vi "iPSset.vi"(7 "Field Rate, T/min":dbl, 8 "error in (no error)":errorcluster, 9 "Target Field, T":dbl, 10 "iPSSetCtrl":T1, 11 "VISA resource name":refnum<visa-resource-name>) -> (0 "error out":errorcluster, 1 "read buffer":string, 2 "number":dbl, 3 "VISA resource name out":refnum<visa-resource-name>)   [LabVIEW 2017]
uses:
  controls/iPSsetCtrl.ctl
  <vilib>/regexp/Match Regular Expression.xnode
panel:
  out "call chain":string[](array[string])
  out "concatenated string 2":string
  out "concatenated string":string
  out "after match":string
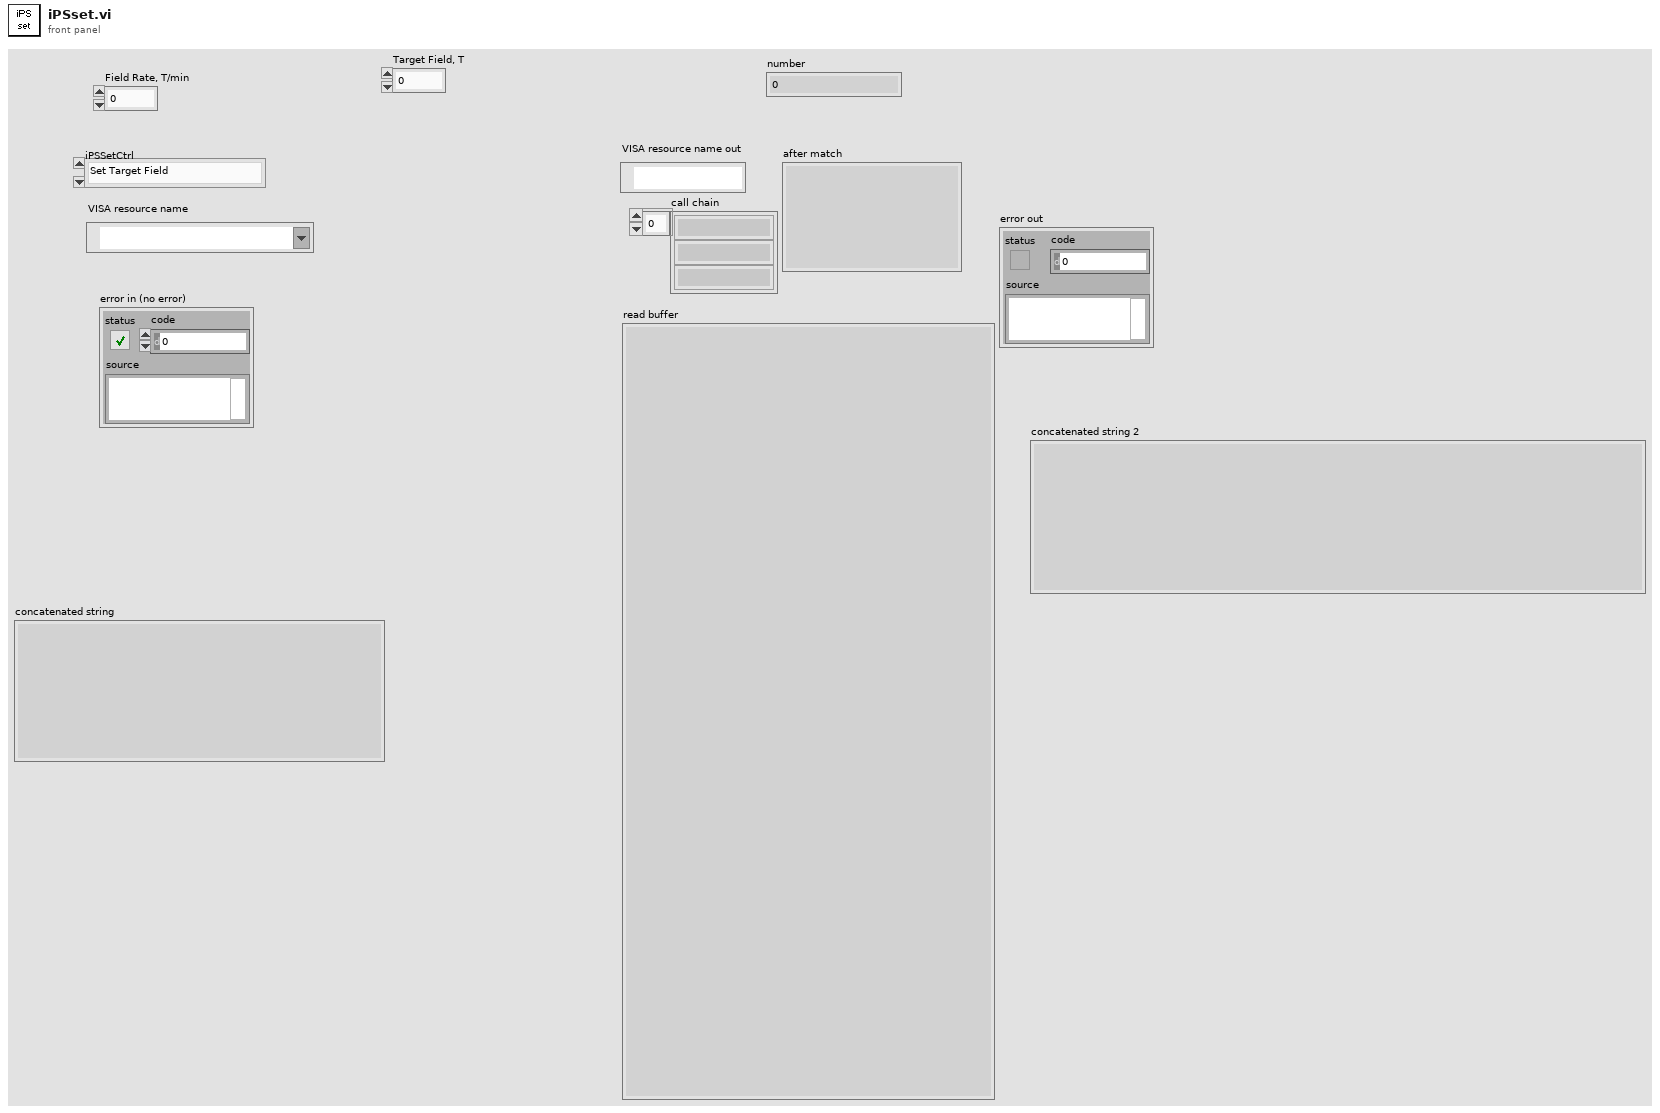
[diagram p1: front panel]
types:
  T1 = typedef "iPSsetCtrl.ctl" = enum16{"Set Target Field", "Set Target Field Rate", "Switch Heater ON", "Switch Heater OFF", "Go to Field", "Go to Zero", "Hold"}
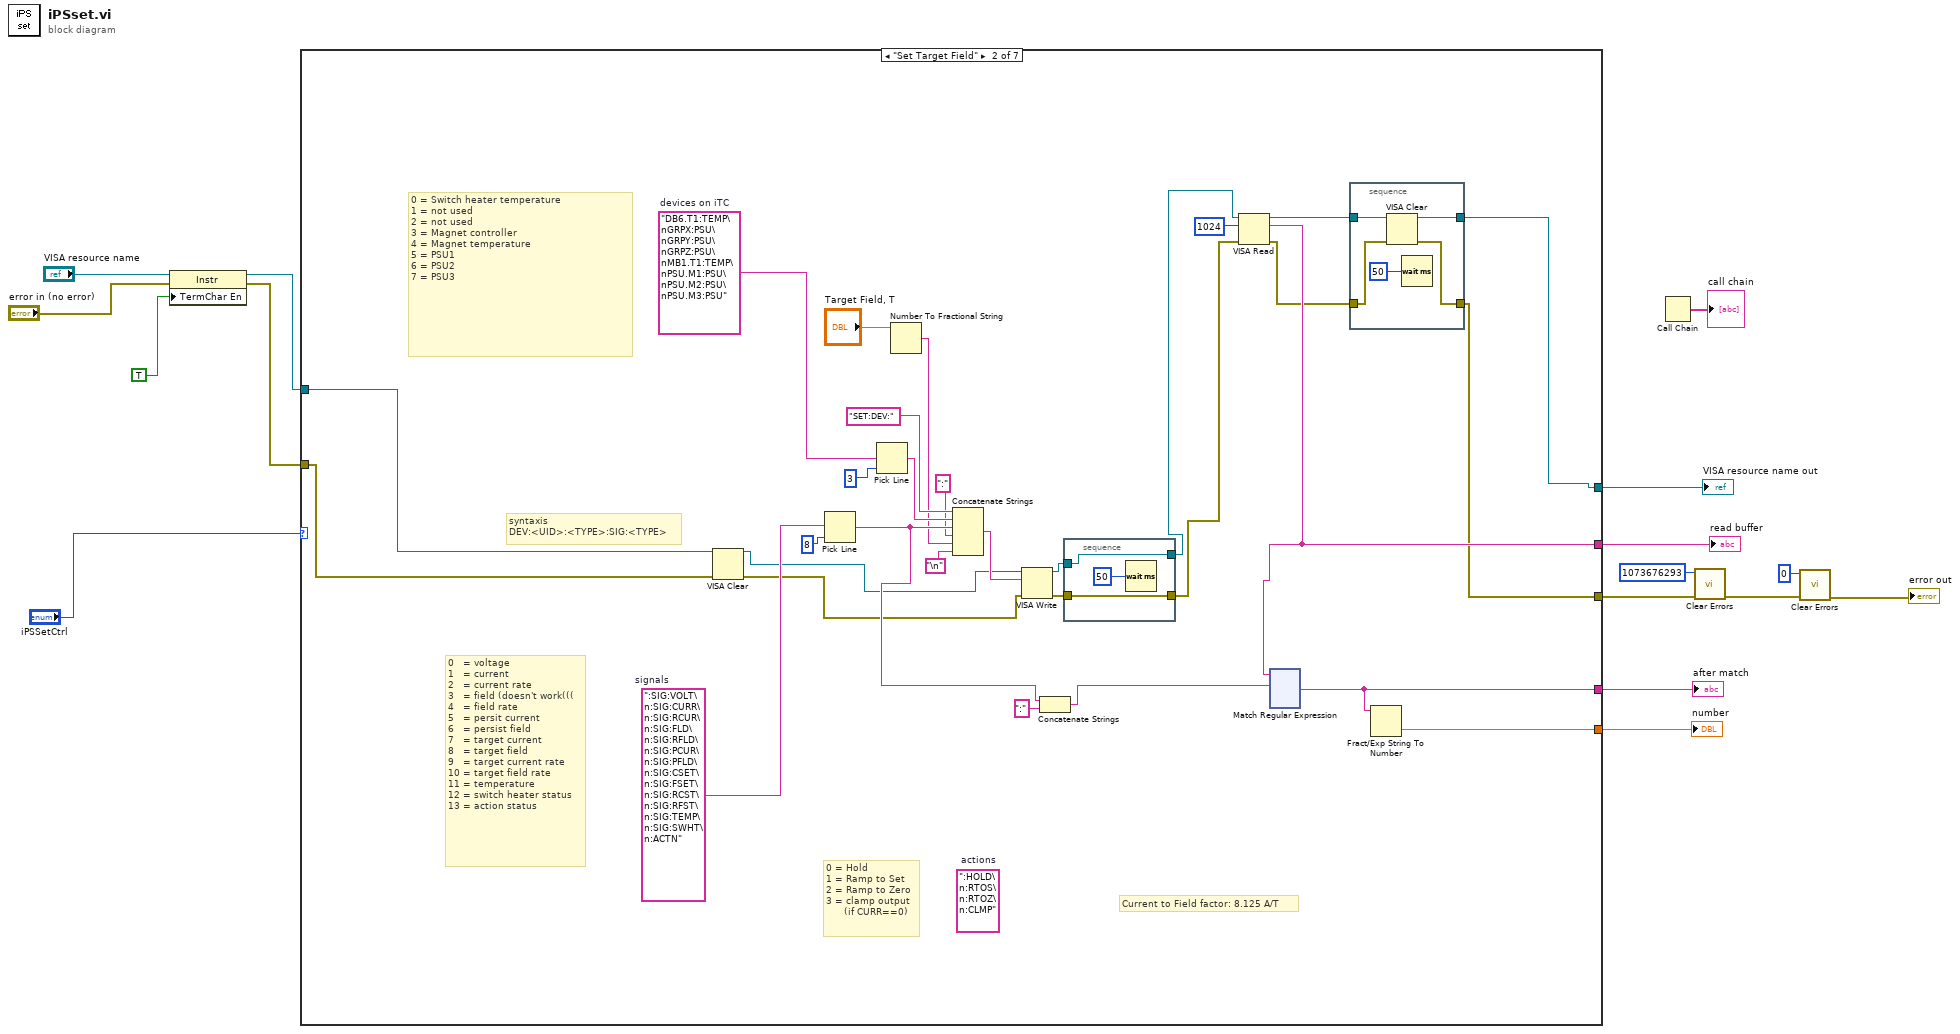
[diagram p0: block diagram]
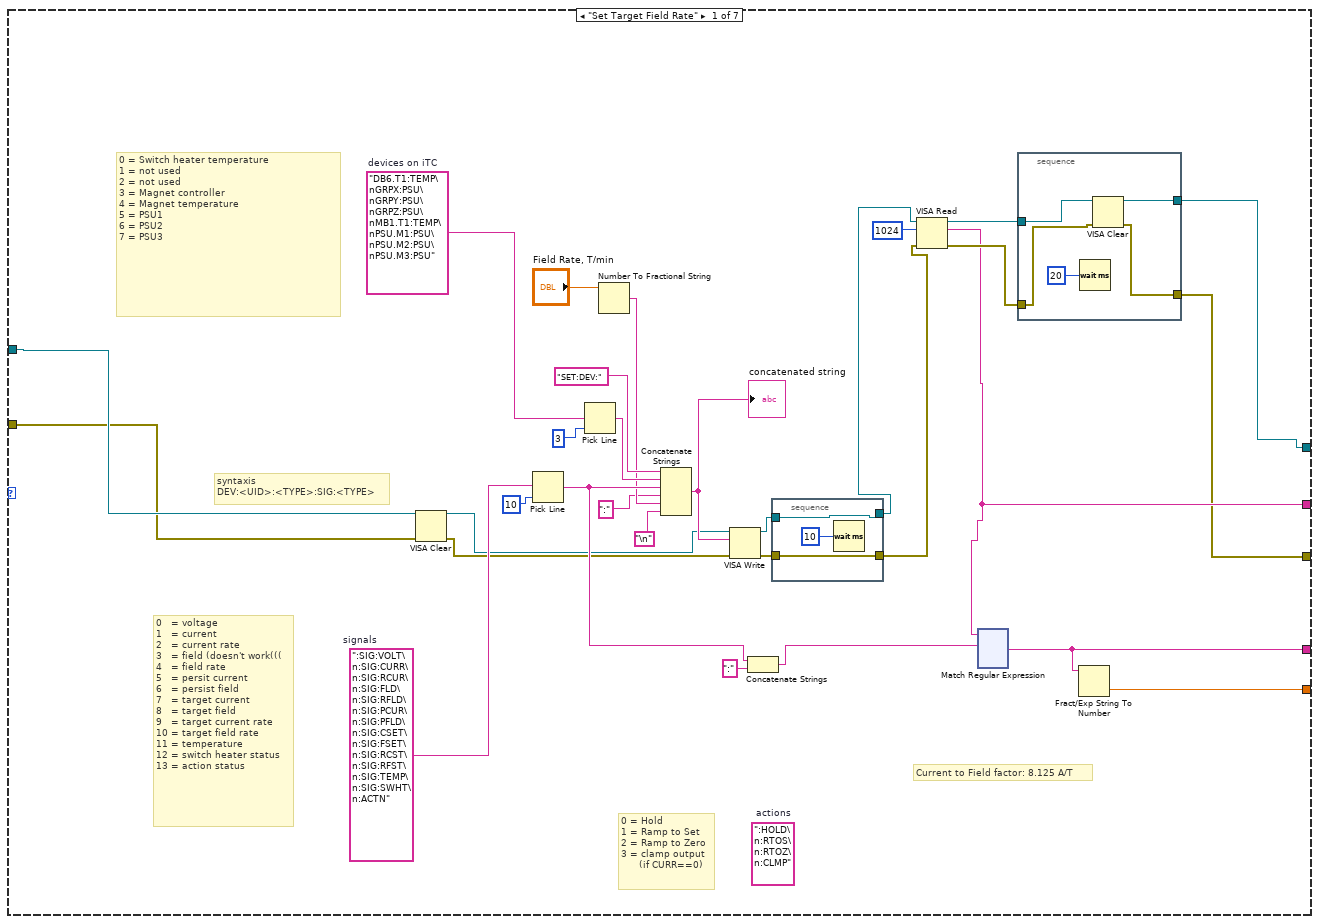
[diagram p2: hidden frame]
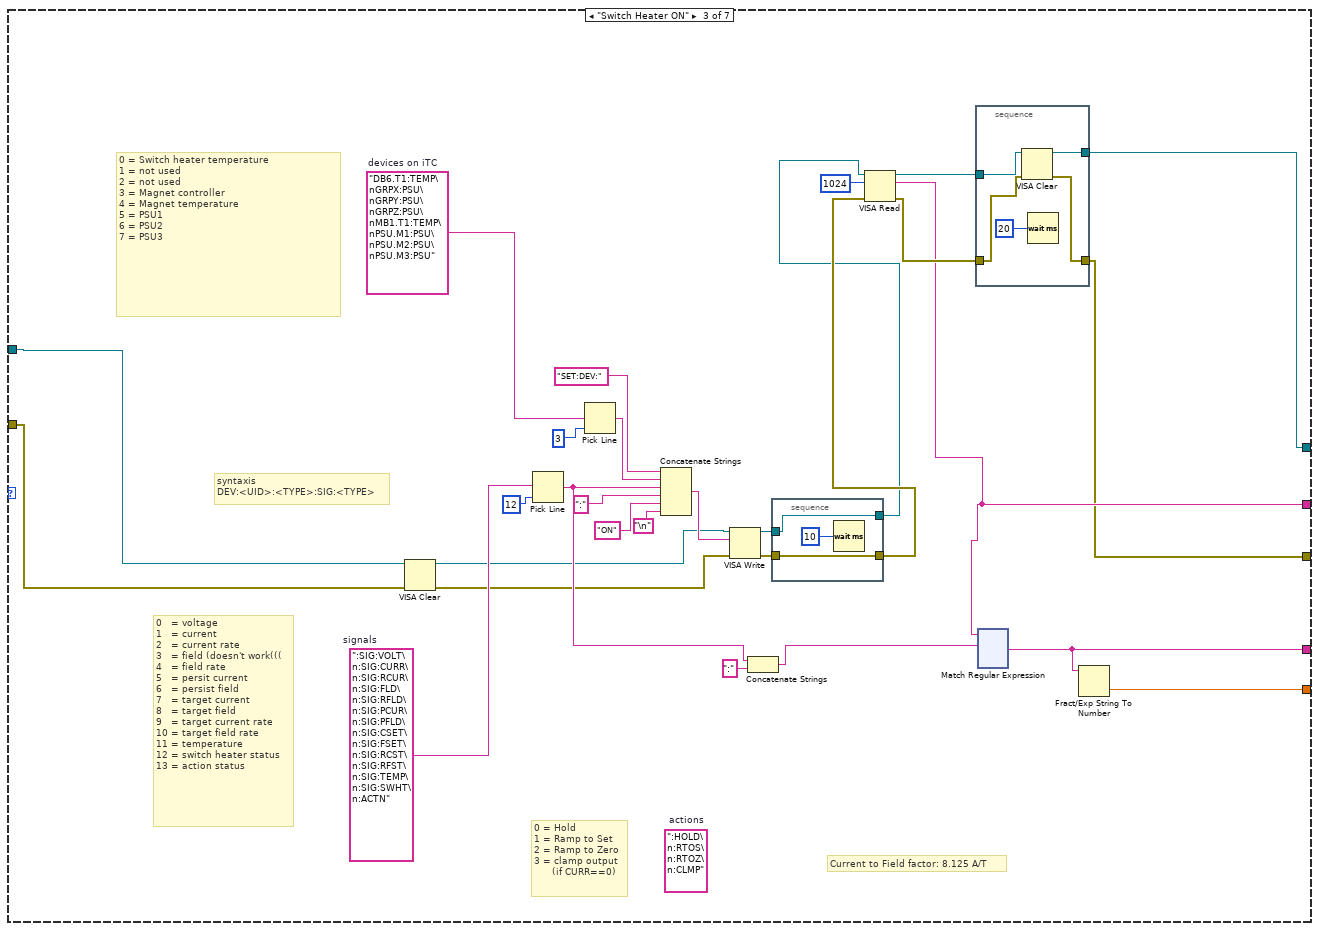
[diagram p3: hidden frame]
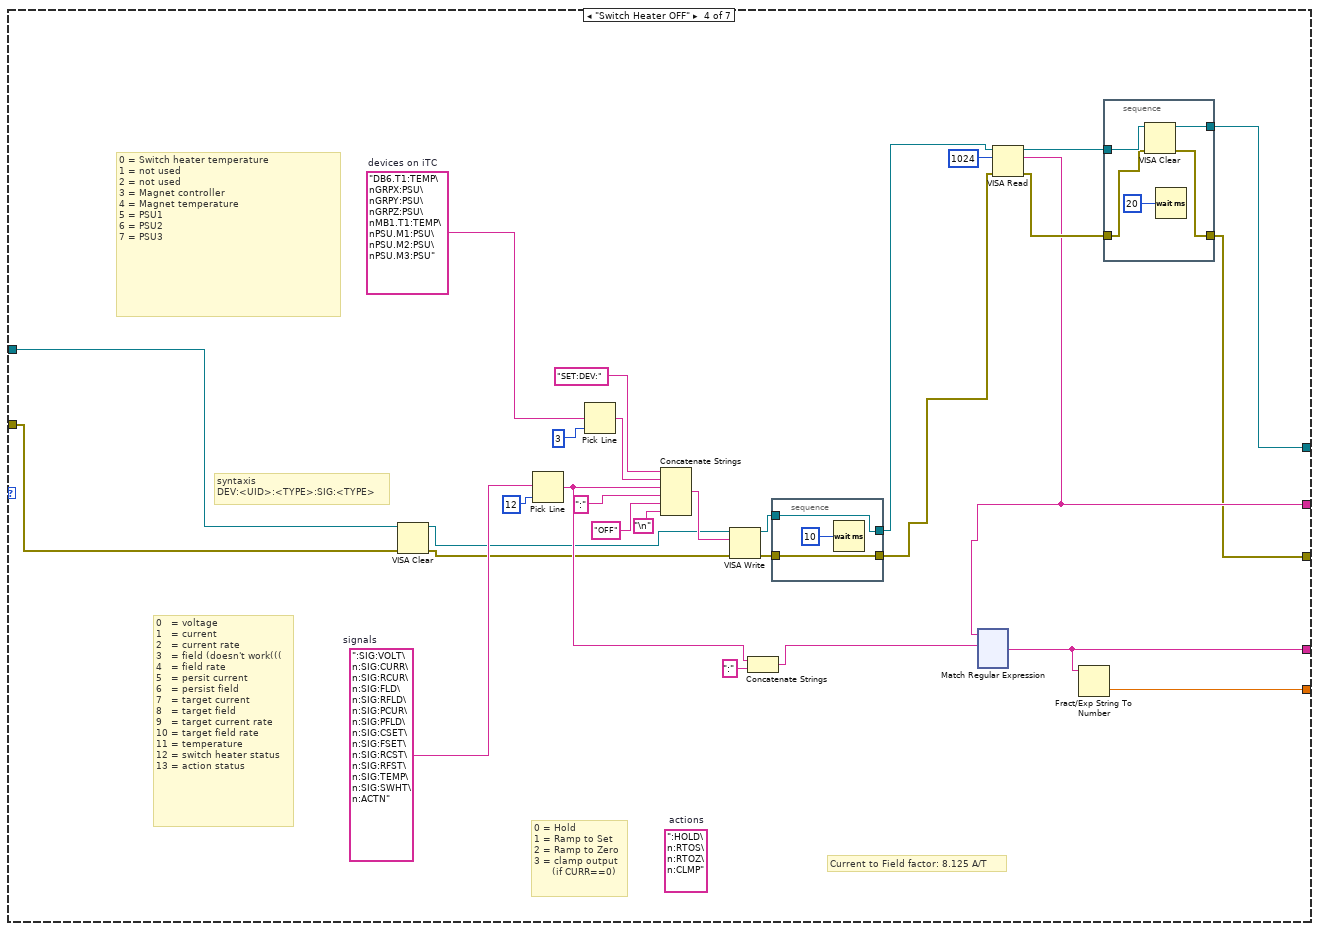
[diagram p4: hidden frame]
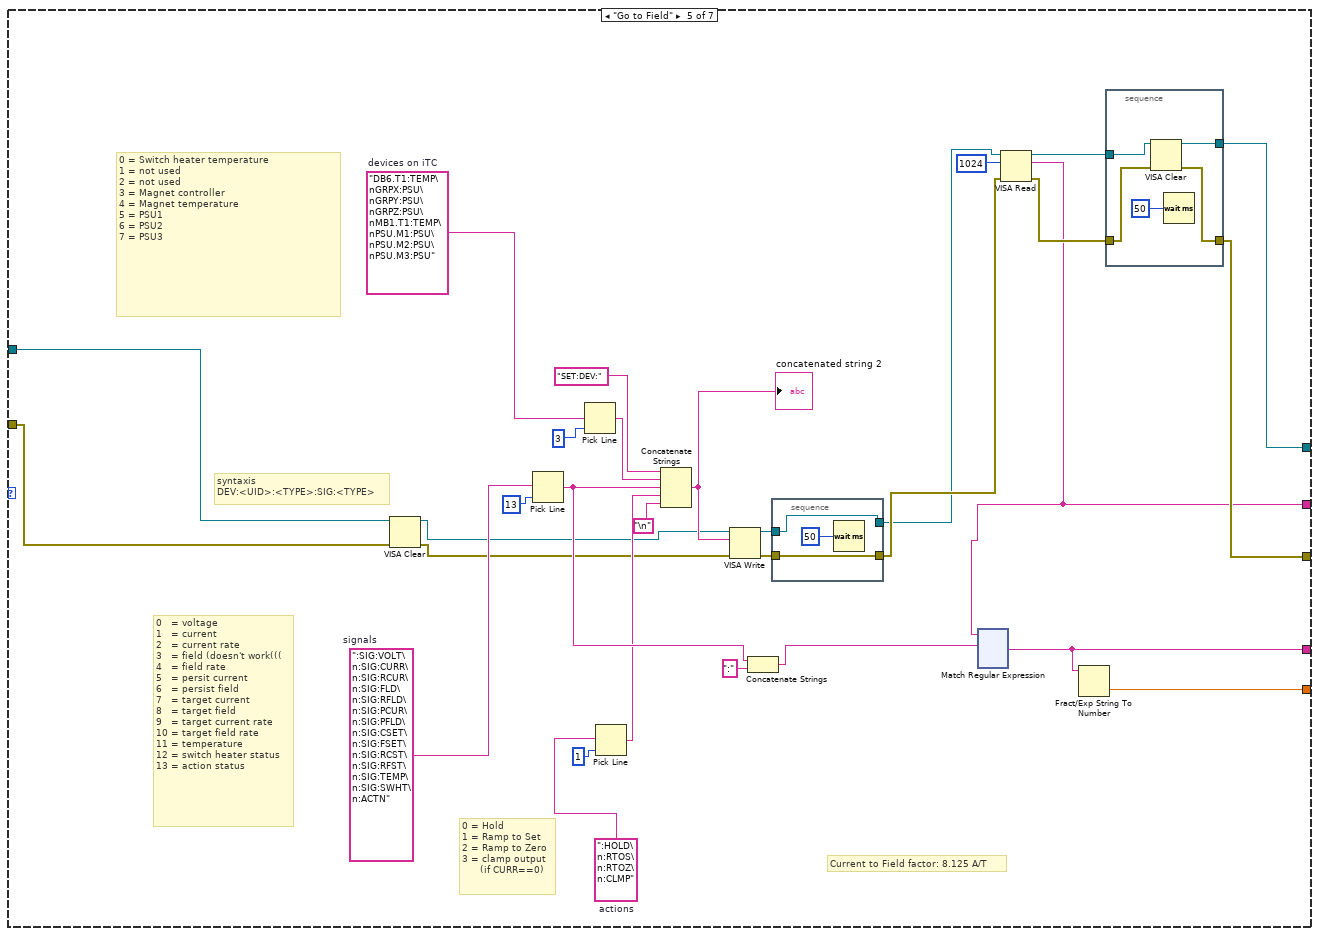
[diagram p5: hidden frame]
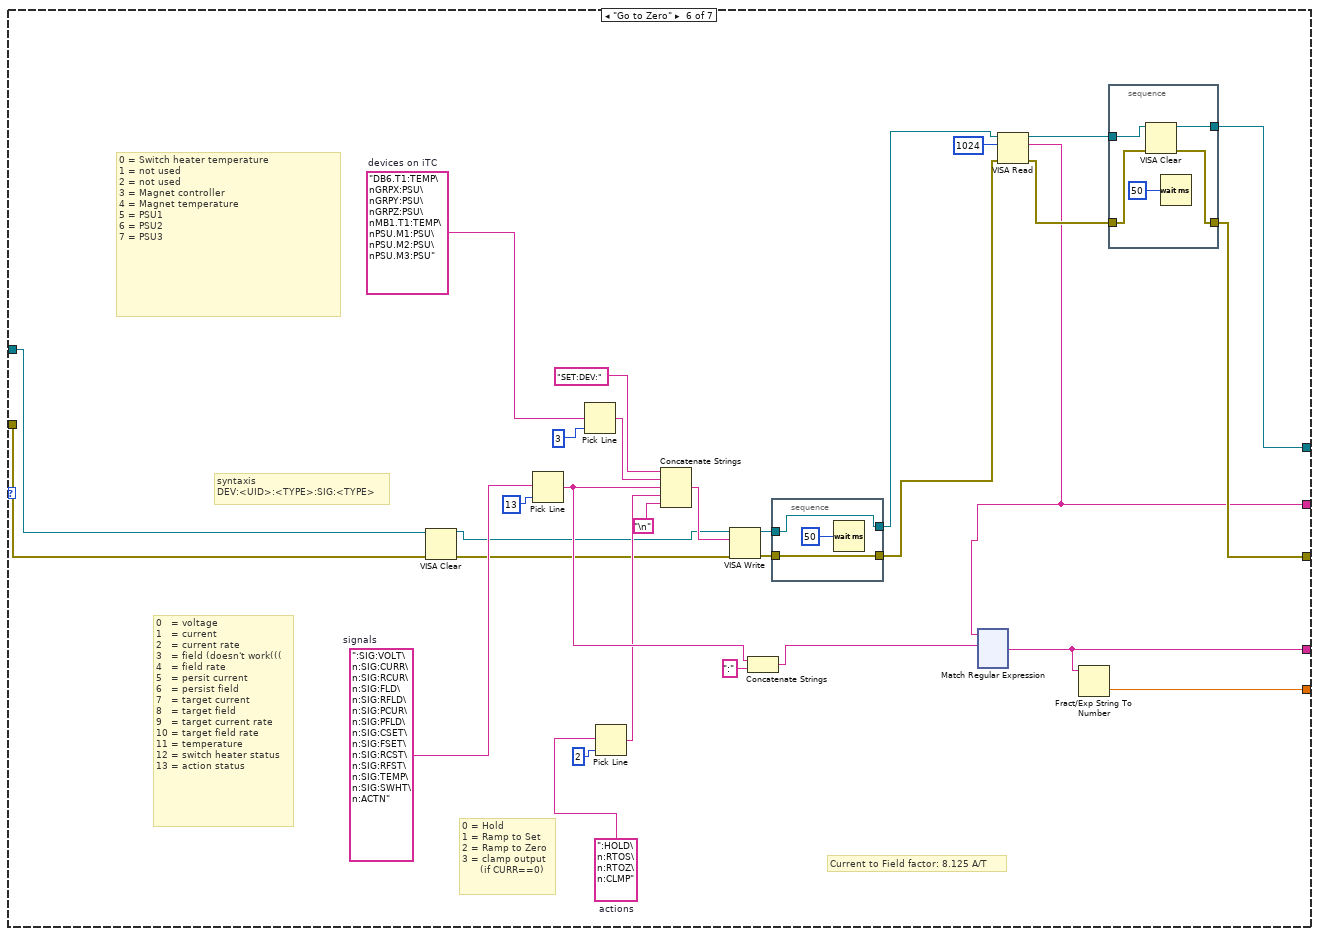
[diagram p6: hidden frame]
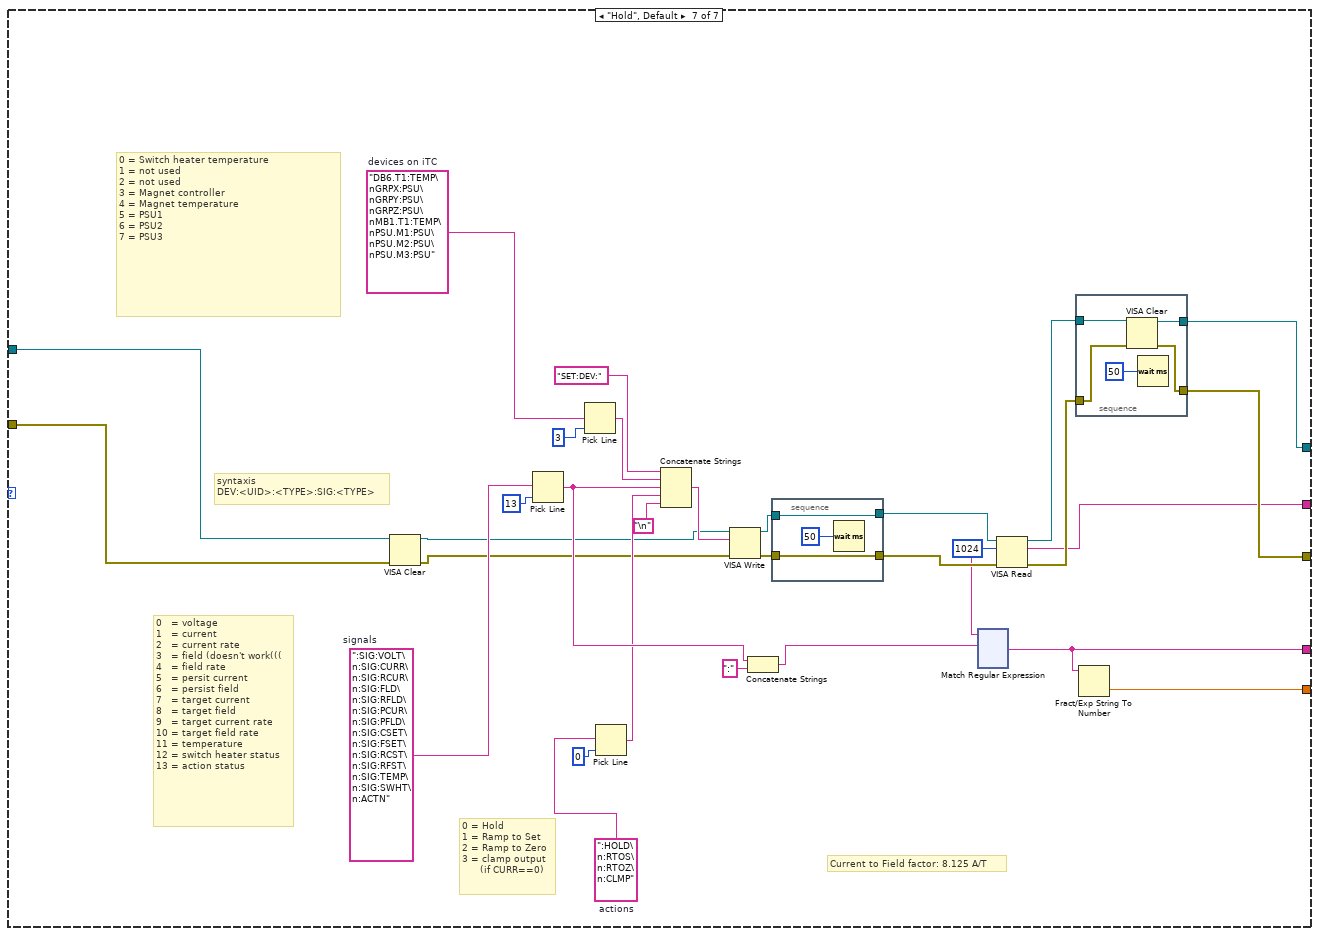
[diagram p7: hidden frame]
diagram:
  n1 = property class="Instr"(reference="VISA resource name", error in="error in (no error)", "TermChar En"=TRUE ("Message Based Settings:Termination Character Enable")) -> (reference out=w10:refnum<visa-resource-name>, error out=w9:errorcluster)
  n2 = case shown="\"Set Target Field\"" "iPSSetCtrl" {
    tunnel: [w25 w174 w323 w471 w621 w770 w918] -> w6
    tunnel: [w19 w168 w317 w465 w613 w763 w911] -> w16
    tunnel: [w26 w176 w324 w472 w620 w768 w917] -> w15
    tunnel: [w36 w185 w333 w481 w630 w779 w928] -> w14
    tunnel: [w35 w184 w332 w480 w629 w778 w927] -> w13
    tunnel: w9 -> [w23 w172 w321 w470 w618 w767 w916]
    tunnel: w10 -> [w24 w173 w322 w467 w616 w764 w913]
    frame "Set Target Field Rate" {
      (unwired) ":HOLD\n:RTOS\n:RTOZ\n:CLMP"  # actions
      w41 = ":SIG:VOLT\n:SIG:CURR\n:SIG:RCUR\n:SIG:FLD\n:SIG:RFLD\n:SIG:PCUR\n:SIG:PFLD\n:SIG:CSET\n:SIG:FSET\n:SIG:RCST\n:SIG:RFST\n:SIG:TEMP\n:SIG:SWHT\n:ACTN"  # signals
      w46 = "DB6.T1:TEMP\nGRPX:PSU\nGRPY:PSU\nGRPZ:PSU\nMB1.T1:TEMP\nPSU.M1:PSU\nPSU.M2:PSU\nPSU.M3:PSU"  # devices on iTC
      # "0 = Hold\n1 = Ramp to Set\n2 = Ramp to Zero\n3 = clamp output\n      (if CURR==0)"
      # "Current to Field factor: 8.125 A/T"
      # "0 = Switch heater temperature\n1 = not used\n2 = not used\n3 = Magnet controller \n4 = Magnet temperature\n5 = PSU1 \n6 = PSU2\n7 = PSU3"
      # "0   = voltage\n1   = current\n2   = current rate\n3   = field (doesn't work(((\n4   = field rate\n5   = persit current\n6   = persist field\n7   = target current\n8   = target field\n9   = target current rate\n10 = target field rate \n11 = temperature\n12 = switch heater status\n13 = action status"
      # "syntaxis\nDEV:<UID>:<TYPE>:SIG:<TYPE>"
      n3 = VISA Clear(VISA resource name=w24, error in (no error)=w23) -> (VISA resource name out=w21:refnum<visa-resource-name>, error out=w22:errorcluster)
      n4 = Pick Line(multi-line string=w41, line index=10) -> (output string=w39:string)  [unwired: 1 in]
      n5 = Pick Line(multi-line string=w46, line index=3) -> (output string=w43:string)  [unwired: 1 in]
      n6 = Number To Fractional String(number="Field Rate, T/min") -> (F-format string=w31:string)  [unwired: 3 in]
      n7 = Concatenate Strings("SET:DEV:" ("write buffer"), w43, w39, ":" ("string"), w31, "\n") -> (w37:string)
      "concatenated string" <- w37
      n8 = VISA Write(VISA resource name=w21, write buffer=w37, error in (no error)=w22) -> (VISA resource name out=w18:refnum<visa-resource-name>, error out=w45:errorcluster)  [unwired: 1 out]
      n9 = Concatenate Strings(w39, ":" ("string")) -> (w38:string)
      n10 = stacked-sequence {
        tunnel: w45 -> [w165]
        tunnel: [w165] -> w27
        tunnel: w18 -> [w163]
        tunnel: [w163] -> w17
        frame #0 {
          n11 = Wait (ms)(milliseconds to wait=u32 10) -> ()  [unwired: 1 out]
        }
      }
      n12 = VISA Read(VISA resource name=w17, byte count=u32 1024, error in (no error)=w27) -> (VISA resource name out=w20:refnum<visa-resource-name>, read buffer=w26:string, error out=w29:errorcluster)  [unwired: 1 out]
      n13 = xnode "Match Regular Expression"("input string"=w26, "regular expression"=w38) -> ("after match"=w36:string)  [unwired: 4 in, 4 out]
      n14 = stacked-sequence {
        tunnel: [w48] -> w25
        tunnel: w29 -> [w47]
        tunnel: w20 -> [w50]
        tunnel: [w49] -> w19
        frame #0 {
          n15 = Wait (ms)(milliseconds to wait=u32 20) -> ()  [unwired: 1 out]
          n16 = VISA Clear(VISA resource name=w50, error in (no error)=w47) -> (VISA resource name out=w49:refnum<visa-resource-name>, error out=w48:errorcluster)
        }
      }
      n17 = Fract/Exp String To Number(string=w36) -> (number=w35:dbl)  [unwired: 3 in, 1 out]
    }
    frame "Set Target Field" {
      (unwired) ":HOLD\n:RTOS\n:RTOZ\n:CLMP"  # actions
      w190 = ":SIG:VOLT\n:SIG:CURR\n:SIG:RCUR\n:SIG:FLD\n:SIG:RFLD\n:SIG:PCUR\n:SIG:PFLD\n:SIG:CSET\n:SIG:FSET\n:SIG:RCST\n:SIG:RFST\n:SIG:TEMP\n:SIG:SWHT\n:ACTN"  # signals
      w195 = "DB6.T1:TEMP\nGRPX:PSU\nGRPY:PSU\nGRPZ:PSU\nMB1.T1:TEMP\nPSU.M1:PSU\nPSU.M2:PSU\nPSU.M3:PSU"  # devices on iTC
      # "0 = Hold\n1 = Ramp to Set\n2 = Ramp to Zero\n3 = clamp output\n      (if CURR==0)"
      # "Current to Field factor: 8.125 A/T"
      # "0 = Switch heater temperature\n1 = not used\n2 = not used\n3 = Magnet controller \n4 = Magnet temperature\n5 = PSU1 \n6 = PSU2\n7 = PSU3"
      # "0   = voltage\n1   = current\n2   = current rate\n3   = field (doesn't work(((\n4   = field rate\n5   = persit current\n6   = persist field\n7   = target current\n8   = target field\n9   = target current rate\n10 = target field rate \n11 = temperature\n12 = switch heater status\n13 = action status"
      # "syntaxis\nDEV:<UID>:<TYPE>:SIG:<TYPE>"
      n18 = VISA Clear(VISA resource name=w173, error in (no error)=w172) -> (VISA resource name out=w170:refnum<visa-resource-name>, error out=w171:errorcluster)
      n19 = Pick Line(multi-line string=w190, line index=8) -> (output string=w188:string)  [unwired: 1 in]
      n20 = Pick Line(multi-line string=w195, line index=3) -> (output string=w192:string)  [unwired: 1 in]
      n21 = Number To Fractional String(number="Target Field, T") -> (F-format string=w180:string)  [unwired: 3 in]
      n22 = Concatenate Strings("SET:DEV:" ("write buffer"), w192, w188, ":" ("string"), w180, "\n") -> (w186:string)
      n23 = VISA Write(VISA resource name=w170, write buffer=w186, error in (no error)=w171) -> (VISA resource name out=w167:refnum<visa-resource-name>, error out=w194:errorcluster)  [unwired: 1 out]
      n24 = Concatenate Strings(w188, ":" ("string")) -> (w187:string)
      n25 = stacked-sequence {
        tunnel: w194 -> [w314]
        tunnel: [w314] -> w177
        tunnel: w167 -> [w312]
        tunnel: [w312] -> w166
        frame #0 {
          n26 = Wait (ms)(milliseconds to wait=u32 50) -> ()  [unwired: 1 out]
        }
      }
      n27 = VISA Read(VISA resource name=w166, byte count=u32 1024, error in (no error)=w177) -> (VISA resource name out=w169:refnum<visa-resource-name>, read buffer=w176:string, error out=w175:errorcluster)  [unwired: 1 out]
      n28 = xnode "Match Regular Expression"("input string"=w176, "regular expression"=w187) -> ("after match"=w185:string)  [unwired: 4 in, 4 out]
      n29 = stacked-sequence {
        tunnel: w175 -> [w198]
        tunnel: [w197] -> w174
        tunnel: w169 -> [w199]
        tunnel: [w196] -> w168
        frame #0 {
          n30 = VISA Clear(VISA resource name=w199, error in (no error)=w198) -> (VISA resource name out=w196:refnum<visa-resource-name>, error out=w197:errorcluster)
          n31 = Wait (ms)(milliseconds to wait=u32 50) -> ()  [unwired: 1 out]
        }
      }
      n32 = Fract/Exp String To Number(string=w185) -> (number=w184:dbl)  [unwired: 3 in, 1 out]
    }
    frame "Switch Heater ON" {
      (unwired) ":HOLD\n:RTOS\n:RTOZ\n:CLMP"  # actions
      w338 = ":SIG:VOLT\n:SIG:CURR\n:SIG:RCUR\n:SIG:FLD\n:SIG:RFLD\n:SIG:PCUR\n:SIG:PFLD\n:SIG:CSET\n:SIG:FSET\n:SIG:RCST\n:SIG:RFST\n:SIG:TEMP\n:SIG:SWHT\n:ACTN"  # signals
      w343 = "DB6.T1:TEMP\nGRPX:PSU\nGRPY:PSU\nGRPZ:PSU\nMB1.T1:TEMP\nPSU.M1:PSU\nPSU.M2:PSU\nPSU.M3:PSU"  # devices on iTC
      # "0 = Hold\n1 = Ramp to Set\n2 = Ramp to Zero\n3 = clamp output\n      (if CURR==0)"
      # "Current to Field factor: 8.125 A/T"
      # "0 = Switch heater temperature\n1 = not used\n2 = not used\n3 = Magnet controller \n4 = Magnet temperature\n5 = PSU1 \n6 = PSU2\n7 = PSU3"
      # "0   = voltage\n1   = current\n2   = current rate\n3   = field (doesn't work(((\n4   = field rate\n5   = persit current\n6   = persist field\n7   = target current\n8   = target field\n9   = target current rate\n10 = target field rate \n11 = temperature\n12 = switch heater status\n13 = action status"
      # "syntaxis\nDEV:<UID>:<TYPE>:SIG:<TYPE>"
      n33 = VISA Clear(VISA resource name=w322, error in (no error)=w321) -> (VISA resource name out=w319:refnum<visa-resource-name>, error out=w320:errorcluster)
      n34 = Pick Line(multi-line string=w338, line index=12) -> (output string=w336:string)  [unwired: 1 in]
      n35 = Pick Line(multi-line string=w343, line index=3) -> (output string=w340:string)  [unwired: 1 in]
      n36 = Concatenate Strings("SET:DEV:" ("write buffer"), w340, w336, ":" ("string"), "ON" ("string"), "\n") -> (w334:string)
      n37 = VISA Write(VISA resource name=w319, write buffer=w334, error in (no error)=w320) -> (VISA resource name out=w315:refnum<visa-resource-name>, error out=w342:errorcluster)  [unwired: 1 out]
      n38 = Concatenate Strings(w336, ":" ("string")) -> (w335:string)
      n39 = stacked-sequence {
        tunnel: w342 -> [w462]
        tunnel: [w462] -> w325
        tunnel: [w460] -> w316
        tunnel: w315 -> [w460]
        frame #0 {
          n40 = Wait (ms)(milliseconds to wait=u32 10) -> ()  [unwired: 1 out]
        }
      }
      n41 = VISA Read(VISA resource name=w316, byte count=u32 1024, error in (no error)=w325) -> (VISA resource name out=w318:refnum<visa-resource-name>, read buffer=w324:string, error out=w326:errorcluster)  [unwired: 1 out]
      n42 = stacked-sequence {
        tunnel: w326 -> [w344]
        tunnel: [w345] -> w323
        tunnel: w318 -> [w347]
        tunnel: [w346] -> w317
        frame #0 {
          n43 = VISA Clear(VISA resource name=w347, error in (no error)=w344) -> (VISA resource name out=w346:refnum<visa-resource-name>, error out=w345:errorcluster)
          n44 = Wait (ms)(milliseconds to wait=u32 20) -> ()  [unwired: 1 out]
        }
      }
      n45 = xnode "Match Regular Expression"("input string"=w324, "regular expression"=w335) -> ("after match"=w333:string)  [unwired: 4 in, 4 out]
      n46 = Fract/Exp String To Number(string=w333) -> (number=w332:dbl)  [unwired: 3 in, 1 out]
    }
    frame "Switch Heater OFF" {
      (unwired) ":HOLD\n:RTOS\n:RTOZ\n:CLMP"  # actions
      w486 = ":SIG:VOLT\n:SIG:CURR\n:SIG:RCUR\n:SIG:FLD\n:SIG:RFLD\n:SIG:PCUR\n:SIG:PFLD\n:SIG:CSET\n:SIG:FSET\n:SIG:RCST\n:SIG:RFST\n:SIG:TEMP\n:SIG:SWHT\n:ACTN"  # signals
      w491 = "DB6.T1:TEMP\nGRPX:PSU\nGRPY:PSU\nGRPZ:PSU\nMB1.T1:TEMP\nPSU.M1:PSU\nPSU.M2:PSU\nPSU.M3:PSU"  # devices on iTC
      # "0 = Hold\n1 = Ramp to Set\n2 = Ramp to Zero\n3 = clamp output\n      (if CURR==0)"
      # "Current to Field factor: 8.125 A/T"
      # "0 = Switch heater temperature\n1 = not used\n2 = not used\n3 = Magnet controller \n4 = Magnet temperature\n5 = PSU1 \n6 = PSU2\n7 = PSU3"
      # "0   = voltage\n1   = current\n2   = current rate\n3   = field (doesn't work(((\n4   = field rate\n5   = persit current\n6   = persist field\n7   = target current\n8   = target field\n9   = target current rate\n10 = target field rate \n11 = temperature\n12 = switch heater status\n13 = action status"
      # "syntaxis\nDEV:<UID>:<TYPE>:SIG:<TYPE>"
      n47 = VISA Clear(VISA resource name=w467, error in (no error)=w470) -> (VISA resource name out=w468:refnum<visa-resource-name>, error out=w469:errorcluster)
      n48 = Pick Line(multi-line string=w486, line index=12) -> (output string=w484:string)  [unwired: 1 in]
      n49 = Pick Line(multi-line string=w491, line index=3) -> (output string=w488:string)  [unwired: 1 in]
      n50 = Concatenate Strings("SET:DEV:" ("write buffer"), w488, w484, ":" ("string"), "OFF" ("string"), "\n") -> (w482:string)
      n51 = VISA Write(VISA resource name=w468, write buffer=w482, error in (no error)=w469) -> (VISA resource name out=w464:refnum<visa-resource-name>, error out=w490:errorcluster)  [unwired: 1 out]
      n52 = Concatenate Strings(w484, ":" ("string")) -> (w483:string)
      n53 = stacked-sequence {
        tunnel: w490 -> [w610]
        tunnel: [w610] -> w473
        tunnel: [w608] -> w463
        tunnel: w464 -> [w608]
        frame #0 {
          n54 = Wait (ms)(milliseconds to wait=u32 10) -> ()  [unwired: 1 out]
        }
      }
      n55 = VISA Read(VISA resource name=w463, byte count=u32 1024, error in (no error)=w473) -> (VISA resource name out=w466:refnum<visa-resource-name>, read buffer=w472:string, error out=w474:errorcluster)  [unwired: 1 out]
      n56 = xnode "Match Regular Expression"("input string"=w472, "regular expression"=w483) -> ("after match"=w481:string)  [unwired: 4 in, 4 out]
      n57 = Fract/Exp String To Number(string=w481) -> (number=w480:dbl)  [unwired: 3 in, 1 out]
      n58 = stacked-sequence {
        tunnel: w474 -> [w492]
        tunnel: [w493] -> w471
        tunnel: w466 -> [w495]
        tunnel: [w494] -> w465
        frame #0 {
          n59 = VISA Clear(VISA resource name=w495, error in (no error)=w492) -> (VISA resource name out=w494:refnum<visa-resource-name>, error out=w493:errorcluster)
          n60 = Wait (ms)(milliseconds to wait=u32 20) -> ()  [unwired: 1 out]
        }
      }
    }
    frame "Go to Field" {
      w625 = ":HOLD\n:RTOS\n:RTOZ\n:CLMP"  # actions
      w635 = ":SIG:VOLT\n:SIG:CURR\n:SIG:RCUR\n:SIG:FLD\n:SIG:RFLD\n:SIG:PCUR\n:SIG:PFLD\n:SIG:CSET\n:SIG:FSET\n:SIG:RCST\n:SIG:RFST\n:SIG:TEMP\n:SIG:SWHT\n:ACTN"  # signals
      w640 = "DB6.T1:TEMP\nGRPX:PSU\nGRPY:PSU\nGRPZ:PSU\nMB1.T1:TEMP\nPSU.M1:PSU\nPSU.M2:PSU\nPSU.M3:PSU"  # devices on iTC
      # "0 = Hold\n1 = Ramp to Set\n2 = Ramp to Zero\n3 = clamp output\n      (if CURR==0)"
      # "Current to Field factor: 8.125 A/T"
      # "0 = Switch heater temperature\n1 = not used\n2 = not used\n3 = Magnet controller \n4 = Magnet temperature\n5 = PSU1 \n6 = PSU2\n7 = PSU3"
      # "0   = voltage\n1   = current\n2   = current rate\n3   = field (doesn't work(((\n4   = field rate\n5   = persit current\n6   = persist field\n7   = target current\n8   = target field\n9   = target current rate\n10 = target field rate \n11 = temperature\n12 = switch heater status\n13 = action status"
      # "syntaxis\nDEV:<UID>:<TYPE>:SIG:<TYPE>"
      n61 = VISA Clear(VISA resource name=w616, error in (no error)=w618) -> (VISA resource name out=w615:refnum<visa-resource-name>, error out=w617:errorcluster)
      n62 = Pick Line(multi-line string=w635, line index=13) -> (output string=w633:string)  [unwired: 1 in]
      n63 = Pick Line(multi-line string=w640, line index=3) -> (output string=w637:string)  [unwired: 1 in]
      n64 = Pick Line(multi-line string=w625, line index=1) -> (output string=w624:string)  [unwired: 1 in]
      n65 = Concatenate Strings("SET:DEV:" ("write buffer"), w637, w633, w624, "\n") -> (w631:string)
      "concatenated string 2" <- w631
      n66 = VISA Write(VISA resource name=w615, write buffer=w631, error in (no error)=w617) -> (VISA resource name out=w612:refnum<visa-resource-name>, error out=w639:errorcluster)  [unwired: 1 out]
      n67 = Concatenate Strings(w633, ":" ("string")) -> (w632:string)
      n68 = stacked-sequence {
        tunnel: w639 -> [w759]
        tunnel: [w759] -> w619
        tunnel: w612 -> [w757]
        tunnel: [w757] -> w611
        frame #0 {
          n69 = Wait (ms)(milliseconds to wait=u32 50) -> ()  [unwired: 1 out]
        }
      }
      n70 = VISA Read(VISA resource name=w611, byte count=u32 1024, error in (no error)=w619) -> (VISA resource name out=w614:refnum<visa-resource-name>, read buffer=w620:string, error out=w622:errorcluster)  [unwired: 1 out]
      n71 = xnode "Match Regular Expression"("input string"=w620, "regular expression"=w632) -> ("after match"=w630:string)  [unwired: 4 in, 4 out]
      n72 = Fract/Exp String To Number(string=w630) -> (number=w629:dbl)  [unwired: 3 in, 1 out]
      n73 = stacked-sequence {
        tunnel: w622 -> [w641]
        tunnel: [w642] -> w621
        tunnel: w614 -> [w644]
        tunnel: [w643] -> w613
        frame #0 {
          n74 = VISA Clear(VISA resource name=w644, error in (no error)=w641) -> (VISA resource name out=w643:refnum<visa-resource-name>, error out=w642:errorcluster)
          n75 = Wait (ms)(milliseconds to wait=u32 50) -> ()  [unwired: 1 out]
        }
      }
    }
    frame "Go to Zero" {
      w774 = ":HOLD\n:RTOS\n:RTOZ\n:CLMP"  # actions
      w784 = ":SIG:VOLT\n:SIG:CURR\n:SIG:RCUR\n:SIG:FLD\n:SIG:RFLD\n:SIG:PCUR\n:SIG:PFLD\n:SIG:CSET\n:SIG:FSET\n:SIG:RCST\n:SIG:RFST\n:SIG:TEMP\n:SIG:SWHT\n:ACTN"  # signals
      w789 = "DB6.T1:TEMP\nGRPX:PSU\nGRPY:PSU\nGRPZ:PSU\nMB1.T1:TEMP\nPSU.M1:PSU\nPSU.M2:PSU\nPSU.M3:PSU"  # devices on iTC
      # "0 = Hold\n1 = Ramp to Set\n2 = Ramp to Zero\n3 = clamp output\n      (if CURR==0)"
      # "Current to Field factor: 8.125 A/T"
      # "0 = Switch heater temperature\n1 = not used\n2 = not used\n3 = Magnet controller \n4 = Magnet temperature\n5 = PSU1 \n6 = PSU2\n7 = PSU3"
      # "0   = voltage\n1   = current\n2   = current rate\n3   = field (doesn't work(((\n4   = field rate\n5   = persit current\n6   = persist field\n7   = target current\n8   = target field\n9   = target current rate\n10 = target field rate \n11 = temperature\n12 = switch heater status\n13 = action status"
      # "syntaxis\nDEV:<UID>:<TYPE>:SIG:<TYPE>"
      n76 = VISA Clear(VISA resource name=w764, error in (no error)=w767) -> (VISA resource name out=w765:refnum<visa-resource-name>, error out=w766:errorcluster)
      n77 = Pick Line(multi-line string=w784, line index=13) -> (output string=w782:string)  [unwired: 1 in]
      n78 = Pick Line(multi-line string=w789, line index=3) -> (output string=w786:string)  [unwired: 1 in]
      n79 = Pick Line(multi-line string=w774, line index=2) -> (output string=w773:string)  [unwired: 1 in]
      n80 = Concatenate Strings("SET:DEV:" ("write buffer"), w786, w782, w773, "\n") -> (w780:string)
      n81 = VISA Write(VISA resource name=w765, write buffer=w780, error in (no error)=w766) -> (VISA resource name out=w761:refnum<visa-resource-name>, error out=w788:errorcluster)  [unwired: 1 out]
      n82 = Concatenate Strings(w782, ":" ("string")) -> (w781:string)
      n83 = stacked-sequence {
        tunnel: w788 -> [w908]
        tunnel: [w908] -> w769
        tunnel: w761 -> [w906]
        tunnel: [w906] -> w760
        frame #0 {
          n84 = Wait (ms)(milliseconds to wait=u32 50) -> ()  [unwired: 1 out]
        }
      }
      n85 = VISA Read(VISA resource name=w760, byte count=u32 1024, error in (no error)=w769) -> (VISA resource name out=w762:refnum<visa-resource-name>, read buffer=w768:string, error out=w771:errorcluster)  [unwired: 1 out]
      n86 = xnode "Match Regular Expression"("input string"=w768, "regular expression"=w781) -> ("after match"=w779:string)  [unwired: 4 in, 4 out]
      n87 = Fract/Exp String To Number(string=w779) -> (number=w778:dbl)  [unwired: 3 in, 1 out]
      n88 = stacked-sequence {
        tunnel: w771 -> [w791]
        tunnel: [w790] -> w770
        tunnel: [w793] -> w763
        tunnel: w762 -> [w792]
        frame #0 {
          n89 = VISA Clear(VISA resource name=w792, error in (no error)=w791) -> (VISA resource name out=w793:refnum<visa-resource-name>, error out=w790:errorcluster)
          n90 = Wait (ms)(milliseconds to wait=u32 50) -> ()  [unwired: 1 out]
        }
      }
    }
    frame "Hold", Default {
      w923 = ":HOLD\n:RTOS\n:RTOZ\n:CLMP"  # actions
      w933 = ":SIG:VOLT\n:SIG:CURR\n:SIG:RCUR\n:SIG:FLD\n:SIG:RFLD\n:SIG:PCUR\n:SIG:PFLD\n:SIG:CSET\n:SIG:FSET\n:SIG:RCST\n:SIG:RFST\n:SIG:TEMP\n:SIG:SWHT\n:ACTN"  # signals
      w938 = "DB6.T1:TEMP\nGRPX:PSU\nGRPY:PSU\nGRPZ:PSU\nMB1.T1:TEMP\nPSU.M1:PSU\nPSU.M2:PSU\nPSU.M3:PSU"  # devices on iTC
      # "0 = Hold\n1 = Ramp to Set\n2 = Ramp to Zero\n3 = clamp output\n      (if CURR==0)"
      # "Current to Field factor: 8.125 A/T"
      # "0 = Switch heater temperature\n1 = not used\n2 = not used\n3 = Magnet controller \n4 = Magnet temperature\n5 = PSU1 \n6 = PSU2\n7 = PSU3"
      # "0   = voltage\n1   = current\n2   = current rate\n3   = field (doesn't work(((\n4   = field rate\n5   = persit current\n6   = persist field\n7   = target current\n8   = target field\n9   = target current rate\n10 = target field rate \n11 = temperature\n12 = switch heater status\n13 = action status"
      # "syntaxis\nDEV:<UID>:<TYPE>:SIG:<TYPE>"
      n91 = VISA Clear(VISA resource name=w913, error in (no error)=w916) -> (VISA resource name out=w914:refnum<visa-resource-name>, error out=w915:errorcluster)
      n92 = Pick Line(multi-line string=w933, line index=13) -> (output string=w931:string)  [unwired: 1 in]
      n93 = Pick Line(multi-line string=w938, line index=3) -> (output string=w935:string)  [unwired: 1 in]
      n94 = Pick Line(multi-line string=w923, line index=0) -> (output string=w922:string)  [unwired: 1 in]
      n95 = Concatenate Strings("SET:DEV:" ("write buffer"), w935, w931, w922, "\n") -> (w929:string)
      n96 = VISA Write(VISA resource name=w914, write buffer=w929, error in (no error)=w915) -> (VISA resource name out=w910:refnum<visa-resource-name>, error out=w937:errorcluster)  [unwired: 1 out]
      n97 = Concatenate Strings(w931, ":" ("string")) -> (w930:string)
      n98 = stacked-sequence {
        tunnel: w937 -> [w1057]
        tunnel: [w1057] -> w920
        tunnel: [w1055] -> w909
        tunnel: w910 -> [w1055]
        frame #0 {
          n99 = Wait (ms)(milliseconds to wait=u32 50) -> ()  [unwired: 1 out]
        }
      }
      n100 = VISA Read(VISA resource name=w909, byte count=u32 1024, error in (no error)=w920) -> (VISA resource name out=w912:refnum<visa-resource-name>, read buffer=w917:string, error out=w919:errorcluster)  [unwired: 1 out]
      n101 = xnode "Match Regular Expression"("input string"=w917, "regular expression"=w930) -> ("after match"=w928:string)  [unwired: 4 in, 4 out]
      n102 = stacked-sequence {
        tunnel: [w940] -> w918
        tunnel: w919 -> [w941]
        tunnel: w912 -> [w942]
        tunnel: [w939] -> w911
        frame #0 {
          n103 = VISA Clear(VISA resource name=w942, error in (no error)=w941) -> (VISA resource name out=w939:refnum<visa-resource-name>, error out=w940:errorcluster)
          n104 = Wait (ms)(milliseconds to wait=u32 50) -> ()  [unwired: 1 out]
        }
      }
      n105 = Fract/Exp String To Number(string=w928) -> (number=w927:dbl)  [unwired: 3 in, 1 out]
    }
  }
  "read buffer" <- w15
  "VISA resource name out" <- w16
  "after match" <- w14
  "number" <- w13
  n106 = Call Chain() -> (call chain=→"call chain":string[])
  n107 = call <vilib>:"Clear Errors.vi"("error in (no error)"=w6, "specific error code to clear (0: all)"=1073676293) -> ("error out"=w3:errorcluster)  [unwired: 4 in, 1 out]
  n108 = call <vilib>:"Clear Errors.vi"("error in (no error)"=w3, "specific error code to clear (0: all)"=0) -> ("error out"=→"error out":errorcluster)  [unwired: 4 in, 1 out]
